vi "901x 9870 DMA Read (Sub).vi"(8 "error in":errorcluster, 9 "Number of bytes":i32, 11 "FPGA In":T1) -> (0 "error out":errorcluster, 1 "Byte Count":u32, 2 "Read Bytes":string, 3 "FPGA Out":T1, 4 "Timed Out":bool, 6 "FPGA Error":errorcluster)   [LabVIEW 2012]
uses:
  <vilib>/rvi/interface/nirviMethod/nirviMethod.xnode
  <vilib>/rvi/interface/nirviReadWriteControl/nirviReadWriteControl.xnode
  FPGA Function.ctl
  901x DMA FPGA Reference.ctl
  <vilib>/rvi/errors/niLvFpgaMergeErrorWithErrorCode.vi
  Program Files (x86)/National Instruments/LabVIEW 2012/examples/CompactRIO/Module Specific/NI 987x/Serial Loopback/VIs/9870 Interface DMA (FPGA).vi
  FPGA Bitfiles/NI-987xSerialLoo_FPGATarget4_9870InterfaceDMA_U4jeboZBP6A.lvbitx
panel:
  # "INPUTS"
  # "OUTPUTS"
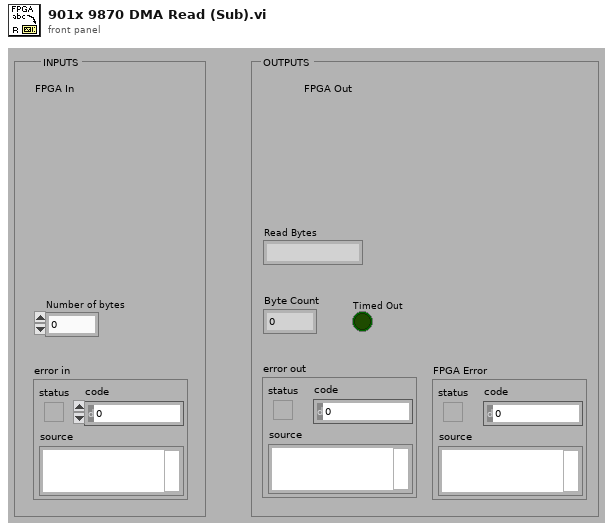
[diagram p1: front panel]
types:
  T1 = typedef "901x DMA FPGA Reference.ctl" = refnum<k20>
  T2 = typedef "FPGA Function.ctl" = enum16{"Do Nothing", "Write", "Read"}
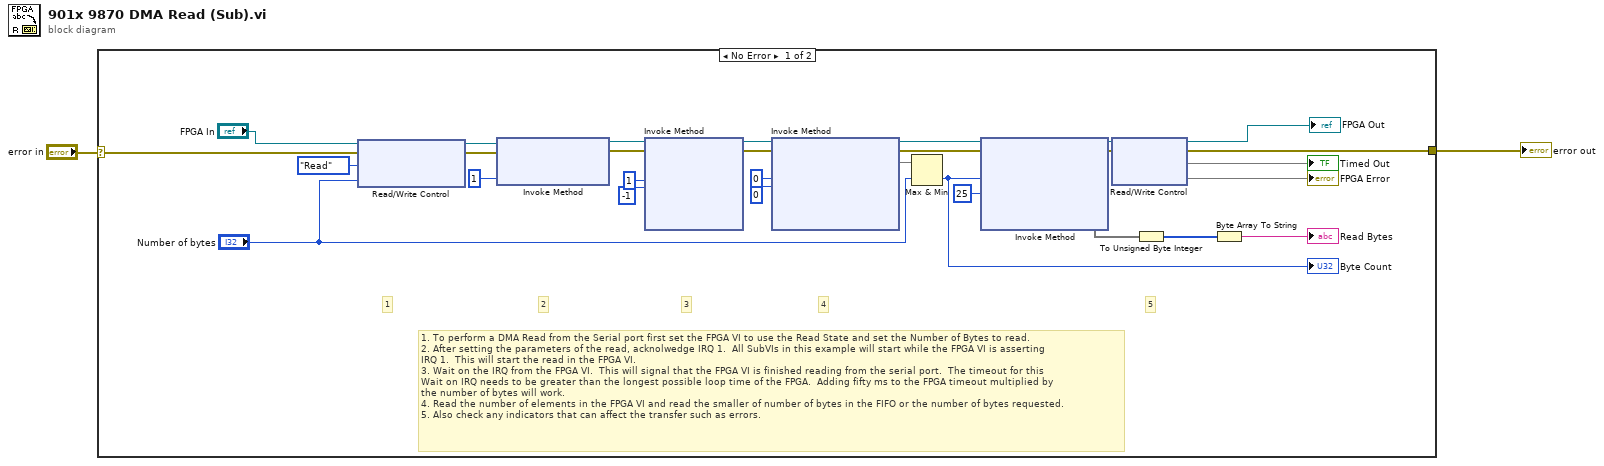
[diagram p0: block diagram]
diagram:
  n1 = case shown="No Error" "error in" {
    selector: "error in" -> [w6 w32]
    tunnel: [w31 w32] -> w2
    frame No Error {
      # "1. To perform a DMA Read from the Serial port first set the FPGA VI to use the Read State and set the Number of Bytes to read.\n2. After setting the parameters of the read, acknolwedge IRQ 1.  All SubVIs in this example will start while the FPGA VI is asserting \nIRQ 1.  This will start the read in the FPGA VI.\n3. Wait on the IRQ from the FPGA VI.  This will signal that the FPGA VI is finished reading from the serial port.  The timeout for this \nWait on IRQ needs to be greater than the longest possible loop time of the FPGA.  Adding fifty ms to the FPGA timeout multiplied by \nthe number of bytes will work.\n4. Read the number of elements in the FPGA VI and read the smaller of number of bytes in the FIFO or the number of bytes requested.\n5. Also check any indicators that can affect the transfer such as errors."
      # "5"
      # "4"
      # "3"
      # "2"
      # "1"
      n2 = xnode "Read/Write Control"("FPGA VI Reference In"="FPGA In", "error in"=w6, "Op Control"=FPGA_Function."Read", "Number of Bytes"="Number of bytes") -> ("FPGA VI Reference Out"=w27:T1, "error out"=w26:errorcluster)
      n3 = xnode "Invoke Method"("FPGA VI Reference In"=w27, "error in"=w26, "IRQ Number(s)"=1) -> ("FPGA VI Reference Out"=w24:T1, "error out"=w23:errorcluster)
      n4 = xnode "Invoke Method"("FPGA VI Reference In"=w24, "error in"=w23, "IRQ Number(s)"=1, "Timeout (ms)"=-1) -> ("FPGA VI Reference Out"=w16:T1, "error out"=w15:errorcluster)  [unwired: 2 out]
      n5 = xnode "Invoke Method"("FPGA VI Reference In"=w16, "error in"=w15, "Number of Elements"=u32 0, "Timeout (ms)"=0) -> ("FPGA VI Reference Out"=w20:T1, "error out"=w19:errorcluster, "Elements Remaining"=w5)  [unwired: 1 out]
      n6 = Max & Min(x=w5, y="Number of bytes") -> (min(x,y)=w11:i32)  [unwired: 1 out]
      "Byte Count" <- w11
      n7 = xnode "Invoke Method"("FPGA VI Reference In"=w20, "error in"=w19, "Number of Elements"=w11, "Timeout (ms)"=25) -> ("FPGA VI Reference Out"=w22:T1, "error out"=w21:errorcluster, "Data"=w9:void[])  [unwired: 1 out]
      n8 = xnode "Read/Write Control"("FPGA VI Reference In"=w22, "error in"=w21) -> ("FPGA VI Reference Out"=→"FPGA Out":T1, "error out"=w31:errorcluster, "Timed Out"=→"Timed Out", "error out"=→"FPGA Error")
      n9 = To Unsigned Byte Integer(number=w9) -> (unsigned 8bit integer=w8:u8[])
      n10 = Byte Array To String(unsigned byte array=w8) -> (string=→"Read Bytes":string)
    }
    frame Error {
    }
  }
  "error out" <- w2
